vi "Match Relaxed Data Type.vi"(6 "Invalid Void Terms?":bool, 8 "error in (no error)":errorcluster, 10 "Data Type to Match":variant, 11 "Array of Data Types":variant[](array[variant])) -> (0 "error out":errorcluster, 3 "Matched Index":i32=-1)   [LabVIEW 2016]
uses:
  <vilib>/Utility/VariantDataType/Type.ctl
  <vilib>/Utility/VariantDataType/VariantType.lvlib
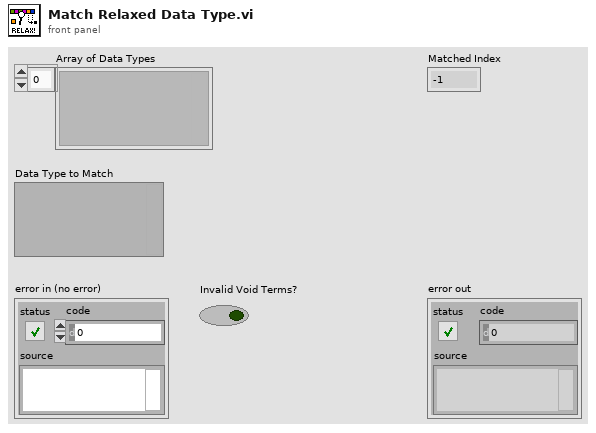
[diagram p1: front panel]
types:
  T1 = typedef "VariantType.lvlib/Type.ctl" = enum8{"Invalid Type", "Void", "I8", "I16", "I32", "I64", "U8", "U16", "U32", "U64", "Single Float", "Double Float", "Extended Float", "Single Complex", "Double Complex", "Extended Complex", "Enum U8", "Enum U16", "Enum U32", "Enum U64", "Single Float With Unit", "Double Float With Unit", "Extended Float With Unit", "Single Complex with Unit", "Double Complex with Unit", "Extended Complex with Unit", "Boolean", "String", "Path", "Picture", "Tag", "Array", "Cluster", "Variant", "LV Variant", "Waveform", "Timestamp", "Digital Waveform", "Digital Data", "ExpressData", "Refnum", "External Data", "VI", "Poly VI", "LabVIEW Class Instance", "Fixed Point"}
  T2 = typedef "VariantType.lvlib/RefnumType.ctl" = enum16{"NotARefnum", "UnknownRefnum", "Generic", "Datalog", "ByteStream", "Device", "Occurence", "TCPNetConnection", "Auto", "Menu", "Imaq", "Hardware", "DataSocket", "Visa", "IVI", "UDPNetConnection", "Notifier", "Queue", "Irda", "EventReg", "DotNet", "UserEvent", "Callback", "UNUSED_EMPTY_POSITION", "BlueToothNetConnection", "LVObjApp", "LVObjVI", "LVObjUnknown", "GenericClass", "UserDefinedRefnumTag", "DataValue", "RT FIFO", "TDMS File"}
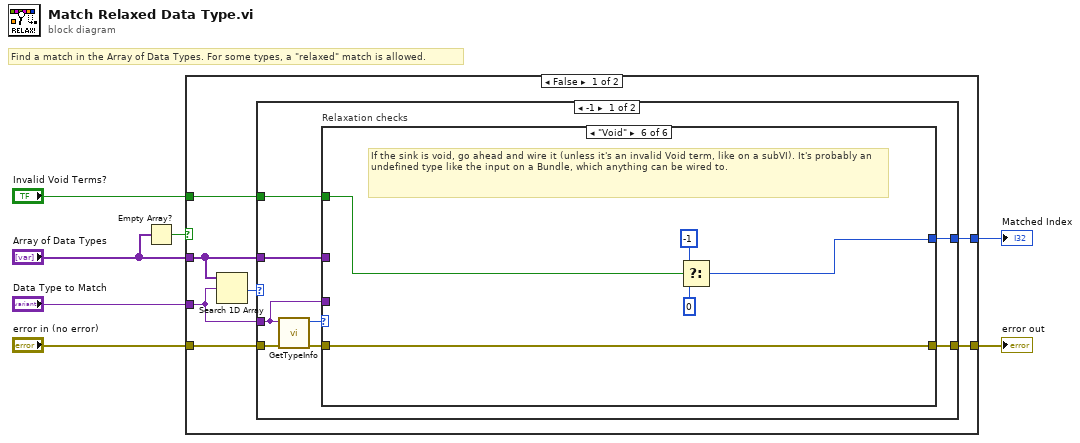
[diagram p0: block diagram]
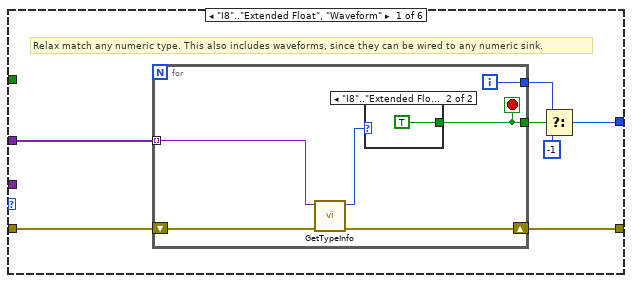
[diagram p2: hidden frame]
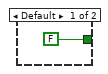
[diagram p3: hidden frame]
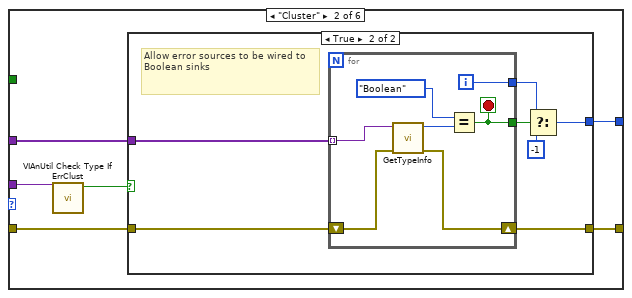
[diagram p4: hidden frame]
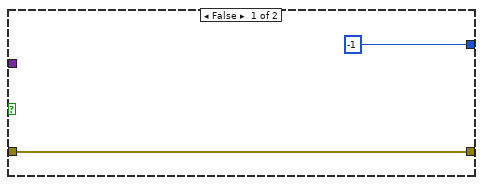
[diagram p5: hidden frame]
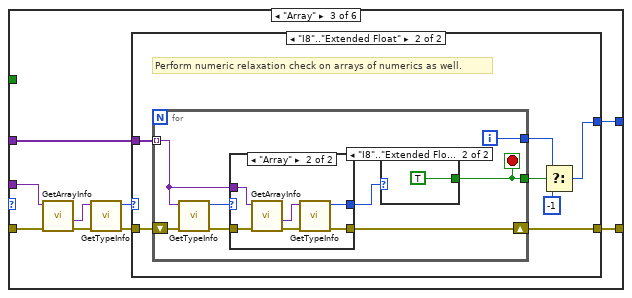
[diagram p6: hidden frame]
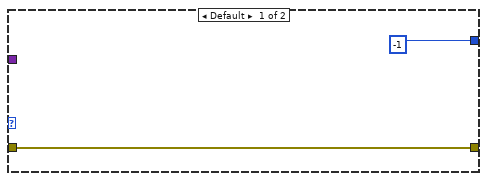
[diagram p7: hidden frame]
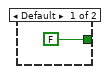
[diagram p9: hidden frame]
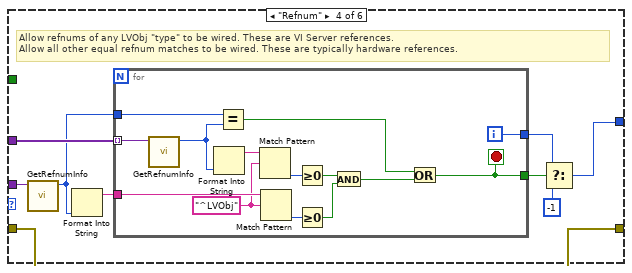
[diagram p10: hidden frame]
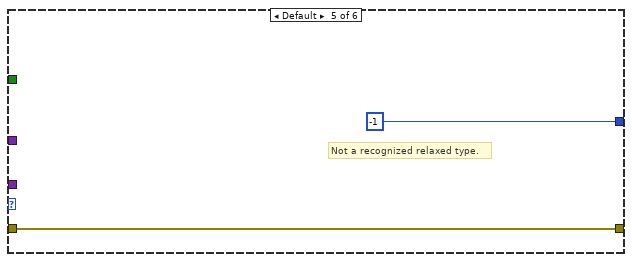
[diagram p11: hidden frame]
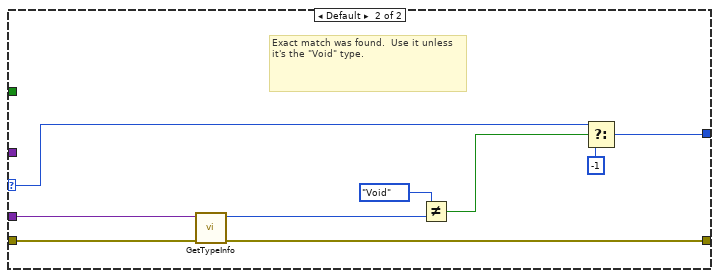
[diagram p12: hidden frame]
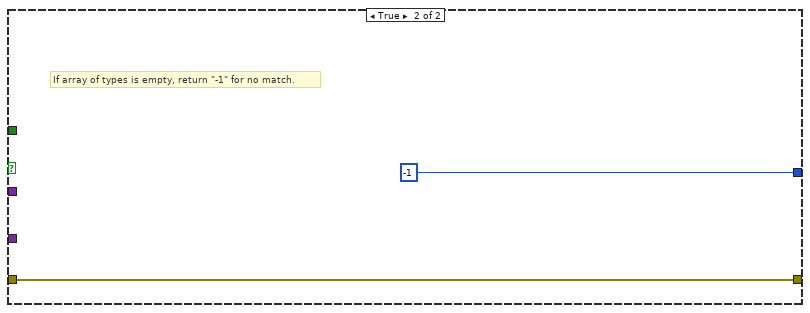
[diagram p13: hidden frame]
diagram:
  # "Find a match in the Array of Data Types. For some types, a \"relaxed\" match is allowed."
  n1 = Empty Array?(array="Array of Data Types") -> (empty?=w2:bool)
  n2 = case shown="False" w2 {
    tunnel: "Data Type to Match" -> [w14 _]
    tunnel: "error in (no error)" -> [w12 w136]
    tunnel: [w11 w136] -> w5
    tunnel: [w10 -1] -> w4
    tunnel: "Array of Data Types" -> [w9 _]
    tunnel: "Invalid Void Terms?" -> [w8 _]
    frame False {
      n3 = Search 1D Array(1D array=w9, element=w14) -> (index of element=w13:i32)  [unwired: 1 in]
      n4 = case shown="-1" w13 {
        selector: w13 -> [_ w128]
        tunnel: [w20 w127] -> w10
        tunnel: w14 -> [w16 w132]
        tunnel: w9 -> [w21 _]
        tunnel: w12 -> [w19 w134]
        tunnel: [w17 w133] -> w11
        tunnel: w8 -> [w15 _]
        frame -1 {
          n5 = call <vilib>:"GetTypeInfo.vi"("error in (no error)"=w19, "Variant"=w16) -> ("error out"=w18:errorcluster, "Type Enum"=w22:T1)  [unwired: 5 in, 3 out]
          n6 = case "Relaxation checks" shown="\"Void\"" w22 {
            tunnel: w21 -> [w29 w43 w68 w104 _ _]
            tunnel: [w25 w42 w67 w101 -1 w122] -> w20
            tunnel: w18 -> [w24 w41 w65 w98 w119 w125]
            tunnel: [w23 w40 w66 w98 w119 w125] -> w17
            tunnel: w16 -> [_ w39 w64 w100 _ _]
            tunnel: w15 -> [_ _ _ _ _ w121]
            frame "I8".."Extended Float", "Waveform" {
              # "Relax match any numeric type. This also includes waveforms, since they can be wired to any numeric sink."
              n7 = for {
                tunnel: w29 -> [w35] mode=indexing
                tunnel: [w33] -> w28
                tunnel: [w32] -> w27
                shift-right: [w30] -> w23
                shift-left: w24 -> [w31]
                i -> [w32]
                stop <- w33 stop-if-true
                n8 = call <vilib>:"GetTypeInfo.vi"("error in (no error)"=w31, "Variant"=w35) -> ("error out"=w30:errorcluster, "Type Enum"=w34:T1)  [unwired: 5 in, 3 out]
                n9 = case shown="\"I8\"..\"Extended Float\", \"Waveform\"" w34 {
                  tunnel: [FALSE TRUE] -> w33
                  frame Default {
                  }
                  frame "I8".."Extended Float", "Waveform" {
                  }
                }
              }
              n10 = Select(t=w27, s=w28, f=-1) -> (s? t:f=w25:i32)
            }
            frame "Cluster" {
              n11 = call <vilib>:"VIAnUtil Check Type If ErrClust.vi"("Data In"=w39) -> ("IsErrClust?"=w38:bool)  [unwired: 9 in, 1 out]
              n12 = case shown="True" w38 {
                tunnel: w43 -> [_ w52]
                tunnel: [-1 w48] -> w42
                tunnel: w41 -> [w45 w47]
                tunnel: [w45 w46] -> w40
                frame False {
                }
                frame True {
                  # "Allow error sources to be wired to Boolean sinks"
                  n13 = for {
                    tunnel: w52 -> [w58] mode=indexing
                    tunnel: [w55] -> w51
                    tunnel: [w59] -> w50
                    shift-right: [w53] -> w46
                    shift-left: w47 -> [w54]
                    i -> [w59]
                    stop <- w55 stop-if-true
                    n14 = call <vilib>:"GetTypeInfo.vi"("error in (no error)"=w54, "Variant"=w58) -> ("error out"=w53:errorcluster, "Type Enum"=w57:T1)  [unwired: 5 in, 3 out]
                    n15 = Equal?(x=Type."Boolean", y=w57) -> (x = y?=w55:bool)
                  }
                  n16 = Select(t=w50, s=w51, f=-1) -> (s? t:f=w48:i32)
                }
              }
            }
            frame "Array" {
              n17 = call <vilib>:"GetArrayInfo.vi"("error in (no error)"=w65, "Variant"=w64) -> ("error out"=w63:errorcluster, "ArrayElement"=w61:variant)  [unwired: 6 in, 2 out]
              n18 = call <vilib>:"GetTypeInfo.vi"("error in (no error)"=w63, "Variant"=w61) -> ("error out"=w62:errorcluster, "Type Enum"=w60:T1)  [unwired: 5 in, 3 out]
              n19 = case shown="\"I8\"..\"Extended Float\"" w60 {
                tunnel: w68 -> [_ w77]
                tunnel: [-1 w73] -> w67
                tunnel: [w70 w72] -> w66
                tunnel: w62 -> [w70 w71]
                frame Default {
                }
                frame "I8".."Extended Float" {
                  # "Perform numeric relaxation check on arrays of numerics as well."
                  n20 = for {
                    tunnel: w77 -> [w78] mode=indexing
                    tunnel: [w85] -> w76
                    tunnel: [w84] -> w75
                    shift-right: [w80] -> w72
                    shift-left: w71 -> [w83]
                    i -> [w84]
                    stop <- w85 stop-if-true
                    n21 = call <vilib>:"GetTypeInfo.vi"("error in (no error)"=w83, "Variant"=w78) -> ("error out"=w82:errorcluster, "Type Enum"=w81:T1)  [unwired: 5 in, 3 out]
                    n22 = case shown="\"Array\"" w81 {
                      selector: w81 -> [w87 _]
                      tunnel: w82 -> [w86 w91]
                      tunnel: [w87 w88] -> w79
                      tunnel: [w86 w92] -> w80
                      tunnel: w78 -> [_ w90]
                      frame Default {
                      }
                      frame "Array" {
                        n23 = call <vilib>:"GetArrayInfo.vi"("error in (no error)"=w91, "Variant"=w90) -> ("error out"=w89:errorcluster, "ArrayElement"=w93:variant)  [unwired: 6 in, 2 out]
                        n24 = call <vilib>:"GetTypeInfo.vi"("error in (no error)"=w89, "Variant"=w93) -> ("error out"=w92:errorcluster, "Type Enum"=w88:T1)  [unwired: 5 in, 3 out]
                      }
                    }
                    n25 = case shown="\"I8\"..\"Extended Float\"" w79 {
                      tunnel: [FALSE TRUE] -> w85
                      frame Default {
                      }
                      frame "I8".."Extended Float" {
                      }
                    }
                  }
                  n26 = Select(t=w75, s=w76, f=-1) -> (s? t:f=w73:i32)
                }
              }
            }
            frame "Refnum" {
              # "Allow refnums of any LVObj \"type\" to be wired. These are VI Server references.\nAllow all other equal refnum matches to be wired. These are typically hardware references."
              n27 = call <vilib>:"GetRefnumInfo.vi"("Variant"=w100) -> ("ReferenceType"=w96:T2)  [unwired: 7 in, 3 out]
              n28 = Format Into String(w96) -> (resulting string=w99:string)  [unwired: 3 in, 1 out]
              n29 = for {
                tunnel: w104 -> [w117] mode=indexing
                tunnel: [w118] -> w103
                tunnel: w99 -> [w116]
                tunnel: [w108] -> w97
                tunnel: w96 -> [w107]
                i -> [w118]
                stop <- w108 stop-if-true
                w113 = "^LVObj" ("regular expression")
                n30 = call <vilib>:"GetRefnumInfo.vi"("Variant"=w117) -> ("ReferenceType"=w106:T2)  [unwired: 7 in, 3 out]
                n31 = Format Into String(w106) -> (resulting string=w114:string)  [unwired: 3 in, 1 out]
                n32 = Equal?(x=w107, y=w106) -> (x = y?=w105:bool)
                n33 = Match Pattern(string=w114, regular expression=w113) -> (offset past match=w112:i32)  [unwired: 1 in, 3 out]
                n34 = Match Pattern(string=w116, regular expression=w113) -> (offset past match=w115:i32)  [unwired: 1 in, 3 out]
                n35 = Greater Or Equal To 0?(x=w112) -> (x >= 0?=w111:bool)
                n36 = Greater Or Equal To 0?(x=w115) -> (x >= 0?=w110:bool)
                n37 = And(x=w111, y=w110) -> (x .and. y?=w109:bool)
                n38 = Or(x=w105, y=w109) -> (x .or. y?=w108:bool)
              }
              n39 = Select(t=w103, s=w97, f=-1) -> (s? t:f=w101:i32)
            }
            frame Default {
              # "Not a recognized relaxed type."
            }
            frame "Void" {
              # "If the sink is void, go ahead and wire it (unless it's an invalid Void term, like on a subVI). It's probably an undefined type like the input on a Bundle, which anything can be wired to."
              n40 = Select(t=-1, s=w121, f=0) -> (s? t:f=w122:i32)
            }
          }
        }
        frame Default {
          # "Exact match was found.  Use it unless it's the \"Void\" type."
          n41 = call <vilib>:"GetTypeInfo.vi"("error in (no error)"=w134, "Variant"=w132) -> ("error out"=w133:errorcluster, "Type Enum"=w131:T1)  [unwired: 5 in, 3 out]
          n42 = Not Equal?(x=Type."Void", y=w131) -> (x != y?=w129:bool)
          n43 = Select(t=w128, s=w129, f=-1) -> (s? t:f=w127:i32)
        }
      }
    }
    frame True {
      # "If array of types is empty, return \"-1\" for no match."
    }
  }
  "Matched Index" <- w4
  "error out" <- w5
